vi "封面信息输入.vi"(8 "错误输入（无错误）":errorcluster caption="error out", 10 "configuration file path":path caption="封面信息路径", 11 "NI_report输入":refnum<class "NI_report.lvclass">) -> (0 "错误输出":errorcluster caption="error out", 1 "版本号":string, 2 "编号":string, 3 "NI_report输出":refnum<class "NI_report.lvclass">, 4 "试验日期":string)   [LabVIEW 2013]
uses:
  <vilib>/Utility/NIReport.llb/NI_report.lvclass
  <vilib>/Utility/config.llb/Read Key (String).vi
  <vilib>/Utility/NIReport.llb/Append Report Text (str wrap).vi
  <vilib>/Utility/config.llb/NI_LVConfig.lvlib
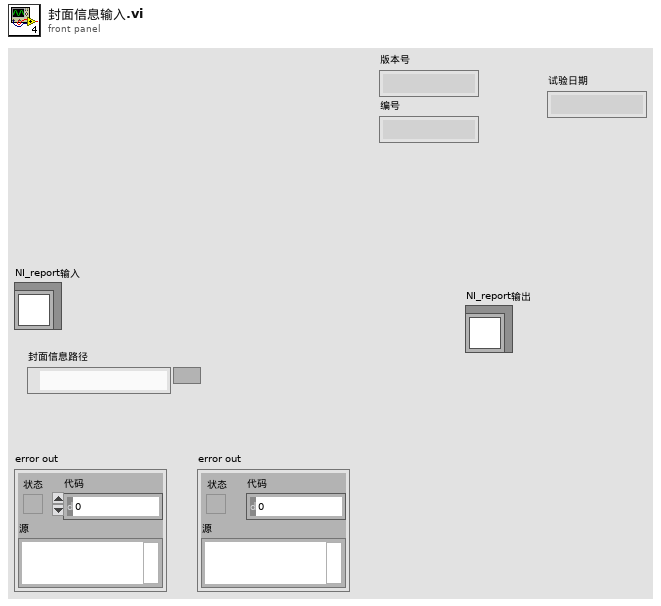
[diagram p1: front panel]
types:
  T1 = cluster{"Charset (-1)":i16, "Weight (-1)":i16, "Name":string, "Size":string}
  T2 = cluster{"Italic":enum16{"Italic Unchanged", "Italic On", "Italic Off"}, "Strike Through":enum16{"Strike Through Unchanged", "Strike Through On", "Strike Through Off"}, "Underline":enum16{"Underline Unchanged", "Underline On", "Underline Off"}, "Bold":enum16{"Bold Unchanged", "Bold On", "Bold Off"}}
  T3 = typedef "NI_LVConfig.lvlib/Config Data RefNum.ctl" = refnum<k1>
  T4 = cluster{"position (excel)":cluster{"row":i32, "column":i32}, "name (excel)":string, "bookmark (word)":string}
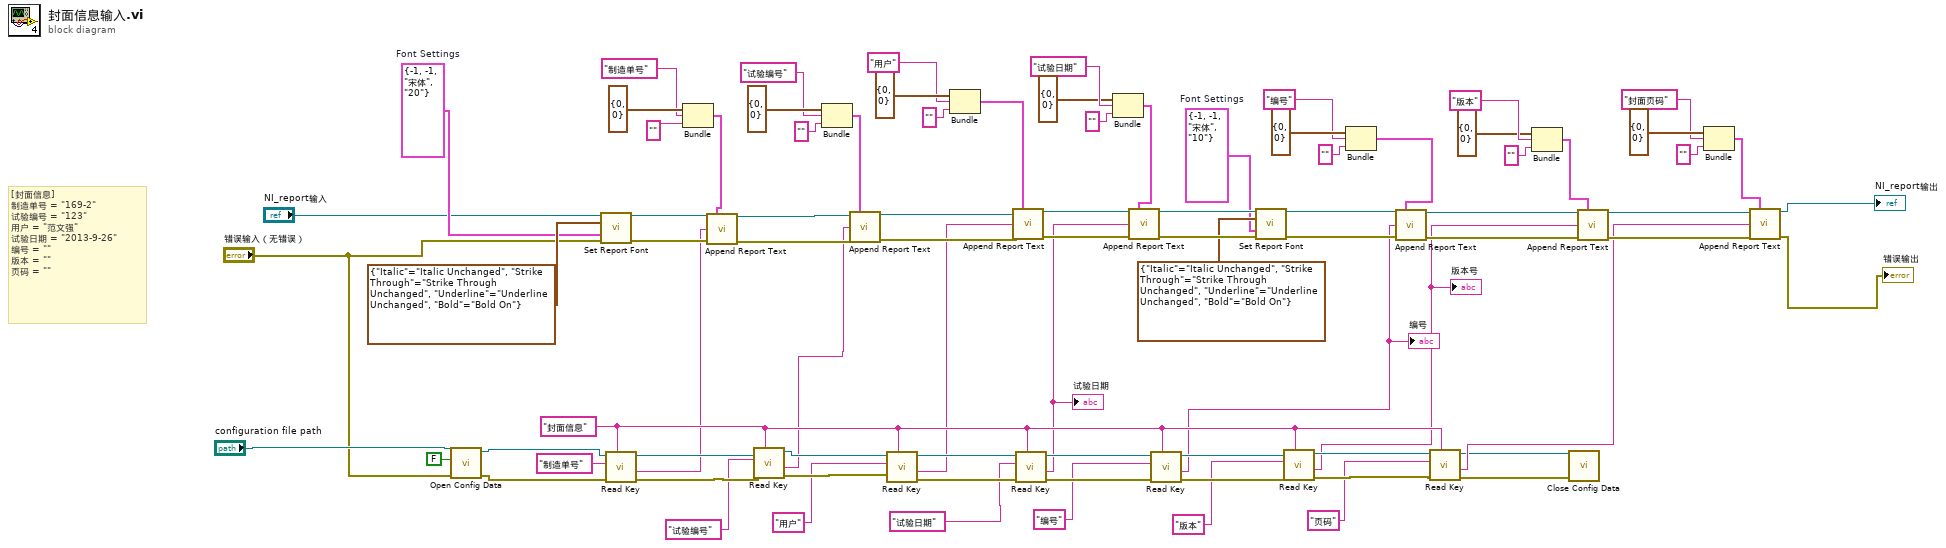
[diagram p0: block diagram]
diagram:
  w28 = T1 {"Charset (-1)"=-1, "Weight (-1)"=-1, "Name"="宋体", "Size"="10"}  # Font Settings
  w32 = "封面信息" ("section")
  w79 = T1 {"Charset (-1)"=-1, "Weight (-1)"=-1, "Name"="宋体", "Size"="20"}  # Font Settings
  # "[封面信息]\n制造单号 = \"169-2\"\n试验编号 = \"123\"\n用户 = \"范文强\"\n试验日期 = \"2013-9-26\"\n编号 = \"\"\n版本 = \"\"\n页码 = \"\""
  n1 = call <vilib>:"Open Config Data.vi"("error in (no error)"="错误输入（无错误）", "create file if necessary (T)"=FALSE, "configuration file path"="configuration file path") -> ("error out"=w52:errorcluster, "refnum"=w53:T3)  [unwired: 6 in, 1 out]
  n2 = call-dynamic "Set Report Font.vi"("report in"="NI_report输入", "text options"=T2 {"Italic"=enum."Italic Unchanged", "Strike Through"=enum."Strike Through Unchanged", "Underline"=enum."Underline Unchanged", "Bold"=enum."Bold On"}, "font settings"=w79, "error in (no error)"="错误输入（无错误）") -> ("report out"=w73:refnum<class "NI_report.lvclass">, "error out"=w74:errorcluster)  [unwired: 9 in, 1 out]
  n3 = call-poly <vilib>:"Read Key.vi"("section"=w32, "error in (no error)"=w52, "key"="制造单号", "refnum"=w53) -> ("error out"=w50:errorcluster, "value"=w2:string, "refnum out"=w49:T3)  [unwired: 4 in, 1 out]
  n4 = Bundle("position (excel)"=cluster{"row":i32, "column":i32} {"row"=0, "column"=0}, "name (excel)"="制造单号", "bookmark (word)"="") -> (w78:T4)  [unwired: 1 in]
  n5 = call-poly <vilib>:"Append Report Text.vi"("report in"=w73, "MS Office parameters"=w78, "text"=w2, "error in (no error)"=w74) -> ("report out"=w84:refnum<class "NI_report.lvclass">, "error out"=w85:errorcluster)  [unwired: 8 in, 2 out]
  n6 = call-poly <vilib>:"Read Key.vi"("section"=w32, "error in (no error)"=w50, "key"="试验编号", "refnum"=w49) -> ("error out"=w48:errorcluster, "value"=w12:string, "refnum out"=w47:T3)  [unwired: 4 in, 1 out]
  n7 = Bundle("position (excel)"=cluster{"row":i32, "column":i32} {"row"=0, "column"=0}, "name (excel)"="试验编号", "bookmark (word)"="") -> (w83:T4)  [unwired: 1 in]
  n8 = call-poly <vilib>:"Append Report Text.vi"("report in"=w84, "MS Office parameters"=w83, "text"=w12, "error in (no error)"=w85) -> ("report out"=w70:refnum<class "NI_report.lvclass">, "error out"=w69:errorcluster)  [unwired: 8 in, 2 out]
  n9 = call-poly <vilib>:"Read Key.vi"("section"=w32, "error in (no error)"=w48, "key"="用户", "refnum"=w47) -> ("error out"=w44:errorcluster, "value"=w11:string, "refnum out"=w43:T3)  [unwired: 4 in, 1 out]
  n10 = Bundle("position (excel)"=cluster{"row":i32, "column":i32} {"row"=0, "column"=0}, "name (excel)"="用户", "bookmark (word)"="") -> (w67:T4)  [unwired: 1 in]
  n11 = call-poly <vilib>:"Append Report Text.vi"("report in"=w70, "MS Office parameters"=w67, "text"=w11, "error in (no error)"=w69) -> ("report out"=w64:refnum<class "NI_report.lvclass">, "error out"=w63:errorcluster)  [unwired: 8 in, 2 out]
  n12 = call-poly <vilib>:"Read Key.vi"("section"=w32, "error in (no error)"=w44, "key"="试验日期", "refnum"=w43) -> ("error out"=w45:errorcluster, "value"=w10:string, "refnum out"=w46:T3)  [unwired: 4 in, 1 out]
  "试验日期" <- w10
  n13 = Bundle("position (excel)"=cluster{"row":i32, "column":i32} {"row"=0, "column"=0}, "name (excel)"="试验日期", "bookmark (word)"="") -> (w59:T4)  [unwired: 1 in]
  n14 = call-poly <vilib>:"Append Report Text.vi"("report in"=w64, "MS Office parameters"=w59, "text"=w10, "error in (no error)"=w63) -> ("report out"=w31:refnum<class "NI_report.lvclass">, "error out"=w30:errorcluster)  [unwired: 8 in, 2 out]
  n15 = call-poly <vilib>:"Read Key.vi"("section"=w32, "error in (no error)"=w45, "key"="编号", "refnum"=w46) -> ("error out"=w39:errorcluster, "value"=w1:string, "refnum out"=w40:T3)  [unwired: 4 in, 1 out]
  "编号" <- w1
  n16 = call-dynamic "Set Report Font.vi"("report in"=w31, "text options"=T2 {"Italic"=enum."Italic Unchanged", "Strike Through"=enum."Strike Through Unchanged", "Underline"=enum."Underline Unchanged", "Bold"=enum."Bold On"}, "font settings"=w28, "error in (no error)"=w30) -> ("report out"=w23:refnum<class "NI_report.lvclass">, "error out"=w22:errorcluster)  [unwired: 9 in, 1 out]
  n17 = call-poly <vilib>:"Read Key.vi"("section"=w32, "error in (no error)"=w39, "key"="版本", "refnum"=w40) -> ("error out"=w42:errorcluster, "value"=w9:string, "refnum out"=w41:T3)  [unwired: 4 in, 1 out]
  "版本号" <- w9
  n18 = Bundle("position (excel)"=cluster{"row":i32, "column":i32} {"row"=0, "column"=0}, "name (excel)"="编号", "bookmark (word)"="") -> (w56:T4)  [unwired: 1 in]
  n19 = call-poly <vilib>:"Append Report Text.vi"("report in"=w23, "MS Office parameters"=w56, "text"=w1, "error in (no error)"=w22) -> ("report out"=w21:refnum<class "NI_report.lvclass">, "error out"=w20:errorcluster)  [unwired: 8 in, 2 out]
  n20 = call-poly <vilib>:"Read Key.vi"("section"=w32, "error in (no error)"=w42, "key"="页码", "refnum"=w41) -> ("error out"=w6:errorcluster, "value"=w8:string, "refnum out"=w7:T3)  [unwired: 4 in, 1 out]
  n21 = Bundle("position (excel)"=cluster{"row":i32, "column":i32} {"row"=0, "column"=0}, "name (excel)"="版本", "bookmark (word)"="") -> (w26:T4)  [unwired: 1 in]
  n22 = call <vilib>:"Close Config Data.vi"("error in (no error)"=w6, "refnum"=w7) -> ()  [unwired: 8 in, 2 out]
  n23 = call-poly <vilib>:"Append Report Text.vi"("report in"=w21, "MS Office parameters"=w26, "text"=w9, "error in (no error)"=w20) -> ("report out"=w14:refnum<class "NI_report.lvclass">, "error out"=w13:errorcluster)  [unwired: 8 in, 2 out]
  n24 = Bundle("position (excel)"=cluster{"row":i32, "column":i32} {"row"=0, "column"=0}, "name (excel)"="封面页码", "bookmark (word)"="") -> (w17:T4)  [unwired: 1 in]
  n25 = call-poly <vilib>:"Append Report Text.vi"("report in"=w14, "MS Office parameters"=w17, "text"=w8, "error in (no error)"=w13) -> ("report out"=→"NI_report输出":refnum<class "NI_report.lvclass">, "error out"=→"错误输出":errorcluster)  [unwired: 8 in, 2 out]
